vi "Global 1 (shooter controls).vi"() -> ()   [LabVIEW 2012]
panel:
  out "ShooterControls":cluster{"ShootNow":bool, "AutoFire":bool}
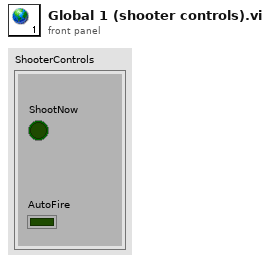
[diagram p1: front panel]
diagram:
